vi "Add Test Information.vi"(8 "error in (no error)":errorcluster, 10 "Test Information":T1, 11 "Report in":refnum<class "Report.lvclass">) -> (0 "error out":errorcluster, 3 "Report out":refnum<class "Report.lvclass">)   [LabVIEW 2015, in "Report.lvclass"]
doc: "This VI takes Test Information and saves it to a local object for writing to disk later."
uses:
  Report.lvclass
  Report Information/Test Information.ctl
  Report.lvclass/Report.ctl
  Report Information/Report Information.lvclass
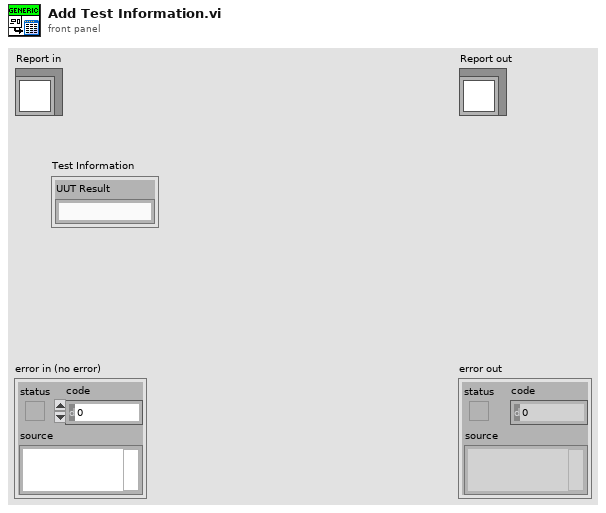
[diagram p1: front panel]
types:
  T1 = typedef "Report Information.lvclass/Test Information.ctl" = cluster{"UUT Result":string}
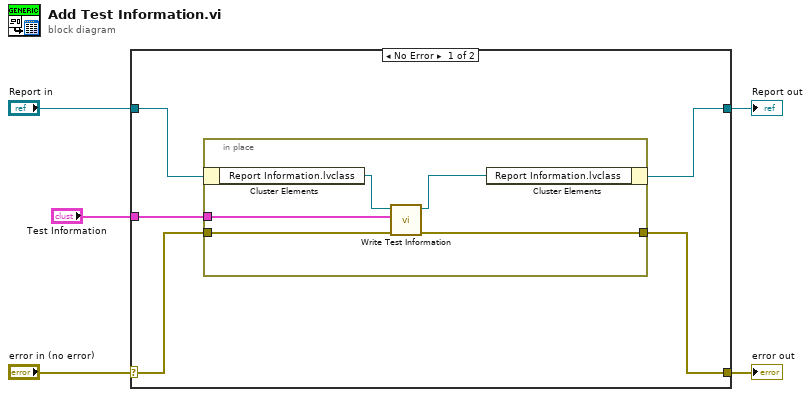
[diagram p0: block diagram]
diagram:
  n1 = case shown="No Error" "error in (no error)" {
    selector: "error in (no error)" -> [w9 w17]
    tunnel: [w8 w17] -> w4
    tunnel: [w7 w16] -> w2
    tunnel: "Report in" -> [w10 w16]
    tunnel: "Test Information" -> [w6 _]
    frame No Error {
      n2 = in-place {
        in-place-border: w9 -> [w15]
        in-place-border: w6 -> [w14]
        in-place-border: [w11] -> w8
        n3 = in-place-cluster #1(w10) -> ("Report Information.lvclass"=w13:refnum<class "Report Information.lvclass">)
        n4 = call-dynamic "Write Test Information.vi"("error in (no error)"=w15, "Test Information"=w14, "Report Information in"=w13) -> ("error out"=w11:errorcluster, "Report Information out"=w12:refnum<class "Report Information.lvclass">)  [unwired: 7 in]
        n5 = in-place-cluster #1("Report Information.lvclass"=w12) -> (w7:refnum<class "Report.lvclass">)
      }
    }
    frame Error {
    }
  }
  "error out" <- w4
  "Report out" <- w2
